vi "daisy.vi"(1 "error in":errorcluster, 2 "USRP RIO device":T1) -> (0 "40 MHz?":bool)   [LabVIEW 2015]
uses:
  <vilib>/userdefined/Silver/nirio_resource_slv.ctl
  PPS_Global_Var.vi
  <vilib>/regexp/Match Regular Expression.xnode
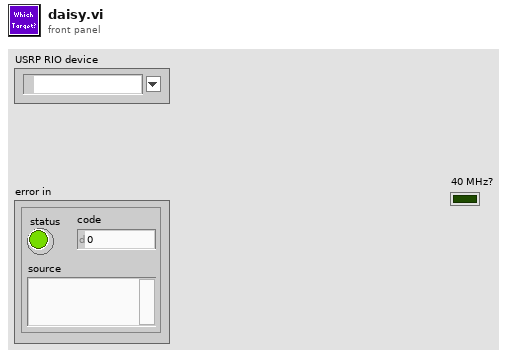
[diagram p1: front panel]
types:
  T1 = typedef "nirio_resource_slv.ctl" = tag
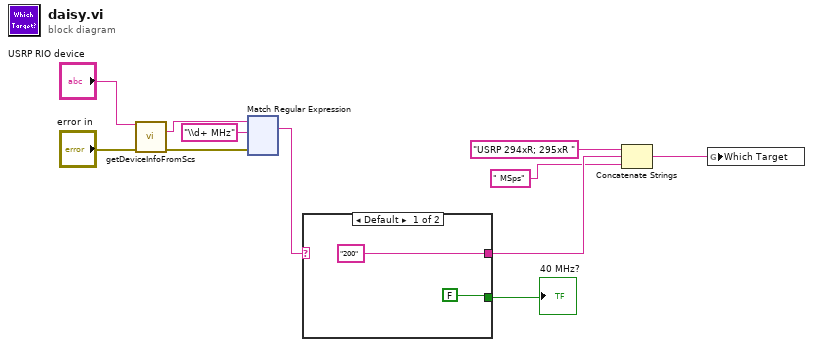
[diagram p0: block diagram]
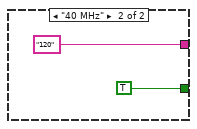
[diagram p2: hidden frame]
diagram:
  n1 = call <vilib>:"getDeviceInfoFromScs.vi"("rio device"="USRP RIO device", "error in"="error in") -> ("product name"=w7:string, "error out"=w8:errorcluster)  [unwired: 9 in, 3 out]
  n2 = xnode "Match Regular Expression"("input string"=w7, "regular expression"="\\d+ MHz", "error in"=w8) -> ("whole match"=w6:string)  [unwired: 3 in, 4 out]
  n3 = case shown="Default" w6 {
    tunnel: ["200" ("format string") "120" ("format string")] -> w3
    tunnel: [FALSE TRUE] -> w5
    frame Default {
    }
    frame "40 MHz" {
    }
  }
  "40 MHz?" <- w5
  n4 = Concatenate Strings("USRP 294xR; 295xR ", w3, " MSps") -> (w1:string)
  n5 = global write "PPS_Global_Var.vi" "Which Target"(w1) -> ()
